vi "Configuration UI.vi"() -> ()   [LabVIEW 2012]
uses:
  cPAS.lvclass
  CRDS/Data/cCRDS Data.lvclass
  Devices/CLAP/CLAP.lvclass
  Reusable/Humidity Control/TEC/TEC Humidity Control.lvclass
  Reusable/PAS/Main/Controls/Laser Modulation.ctl
  Interface/Controls/pasLasCtl.ctl
  Interface/Controls/PAS_MFC_SP.ctl
  Interface/Controls/pasCellTEC.ctl
  Interface/Controls/pasTECen.ctl
  FPGA/Controls/FPGAConfig.ctl
panel:
  in  "ACpow":T1
  in  "pages":enum32{"general", "pas", "crds"}(tab)
  in  "pasTECEn":T2 caption="Enable TECs"
  in  "pasTcell":T3 caption="Temperature \n (degC)"
  in  "pasFlows":T4 caption="Flow Rate Setpoint (LPM)" {"Cell 5" min=0 max=5; "Cell 4" min=0 max=5; "Cell 3" min=0 max=5; "Cell 2" min=0 max=5; "Cell 1" min=0 max=5}
  in  "pasTteSP":sgl caption="TEC Temperature \nSetpoint (degC)" format="%#.2f"
  in  "pasLasCtl":T5 caption="Laser Control" {"Laser Output"."Span"."ch 5" min=0 max=20; "Laser Output"."Span"."ch 4" min=0 max=20; "Laser Output"."Span"."ch 3" min=0 max=20; "Laser Output"."Span"."ch 2" min=0 max=20; "Laser Output"."Span"."ch 1" min=0 max=20; "f0"."Cell 1" min=0 max=2000 step=1; "f0"."Cell 2" min=0 max=2000 step=1; "f0"."Cell 3" min=0 max=2000 step=1; "f0"."Cell 4" min=0 max=2000 step=1; "f0"."Cell 5" min=0 max=2000 step=1}
  # "TEC Temperature Control"
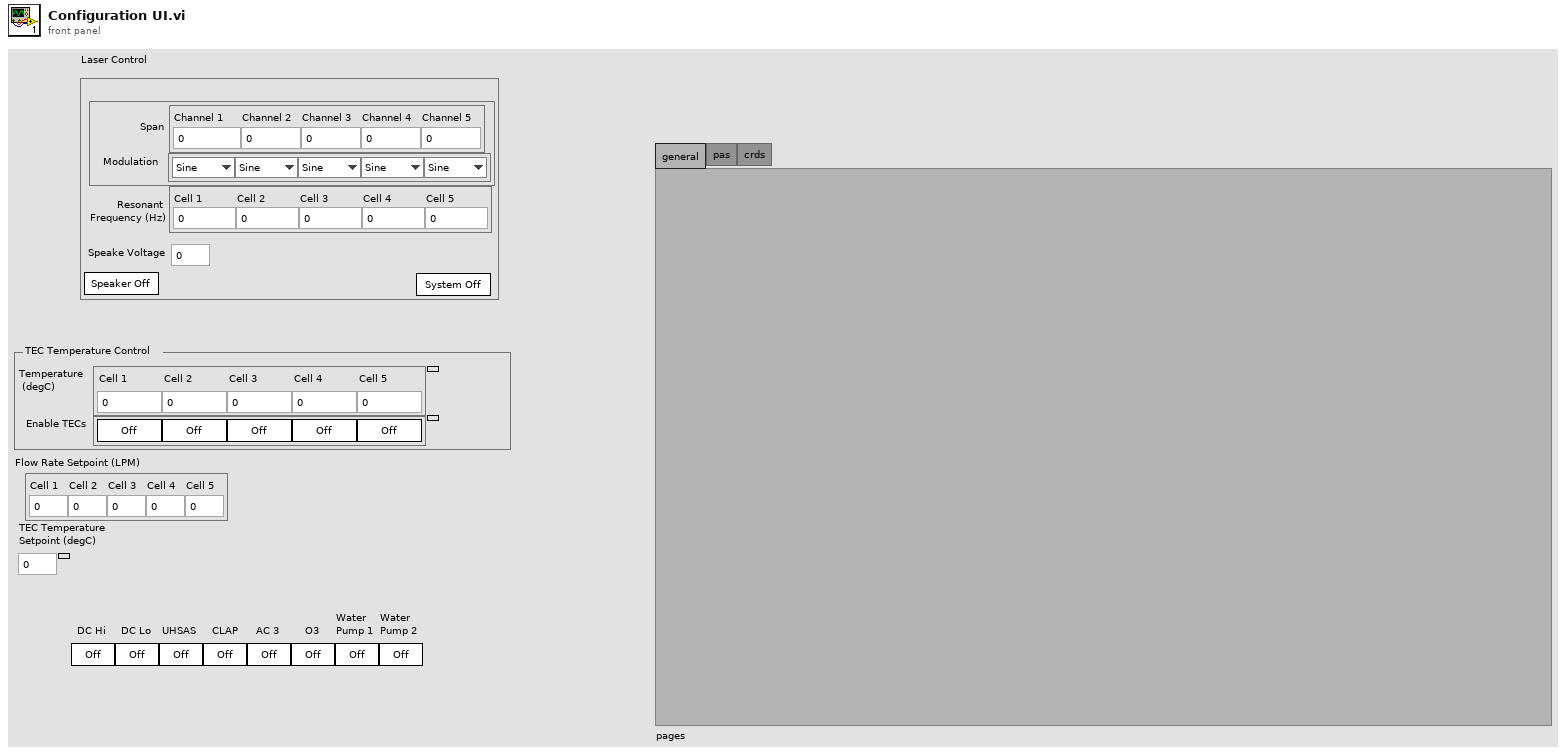
[diagram p1: front panel]
types:
  T1 = cluster{"ac1 2":bool, "ac1 3":bool, "ac1":bool, "ac2":bool, "ac3":bool, "O3":bool, "wp1":bool, "wp2":bool}
  T2 = typedef "pasTECen.ctl" = cluster{"Cell 1":bool, "Cell 2":bool, "Cell 3":bool, "Cell 4":bool, "Cell 5":bool}
  T3 = typedef "pasCellTEC.ctl" = cluster{"Cell 1":sgl, "Cell 2":sgl, "Cell 3":sgl, "Cell 4":sgl, "Cell 5":sgl}
  T4 = typedef "PAS_MFC_SP.ctl" = cluster{"Cell 1":sgl, "Cell 2":sgl, "Cell 3":sgl, "Cell 4":sgl, "Cell 5":sgl}
  T5 = typedef "pasLasCtl.ctl" = cluster{"Laser Output":T6, "f0":cluster{"Cell 1":sgl, "Cell 2":sgl, "Cell 3":sgl, "Cell 4":sgl, "Cell 5":sgl}, "drive":bool, "lasSysPow":bool, "Speake Voltage":dbl}
  T6 = typedef "FPGAConfig.ctl" = cluster{"Span":cluster{"ch 1":sgl, "ch 2":sgl, "ch 3":sgl, "ch 4":sgl, "ch 5":sgl}, "mod":cluster{"ch 1":T7, "ch 2":T7, "ch 3":T7, "ch 4":T7, "ch 5":T7}}
  T7 = typedef "Laser Modulation.ctl" = enum8{"Sine", "Square"}
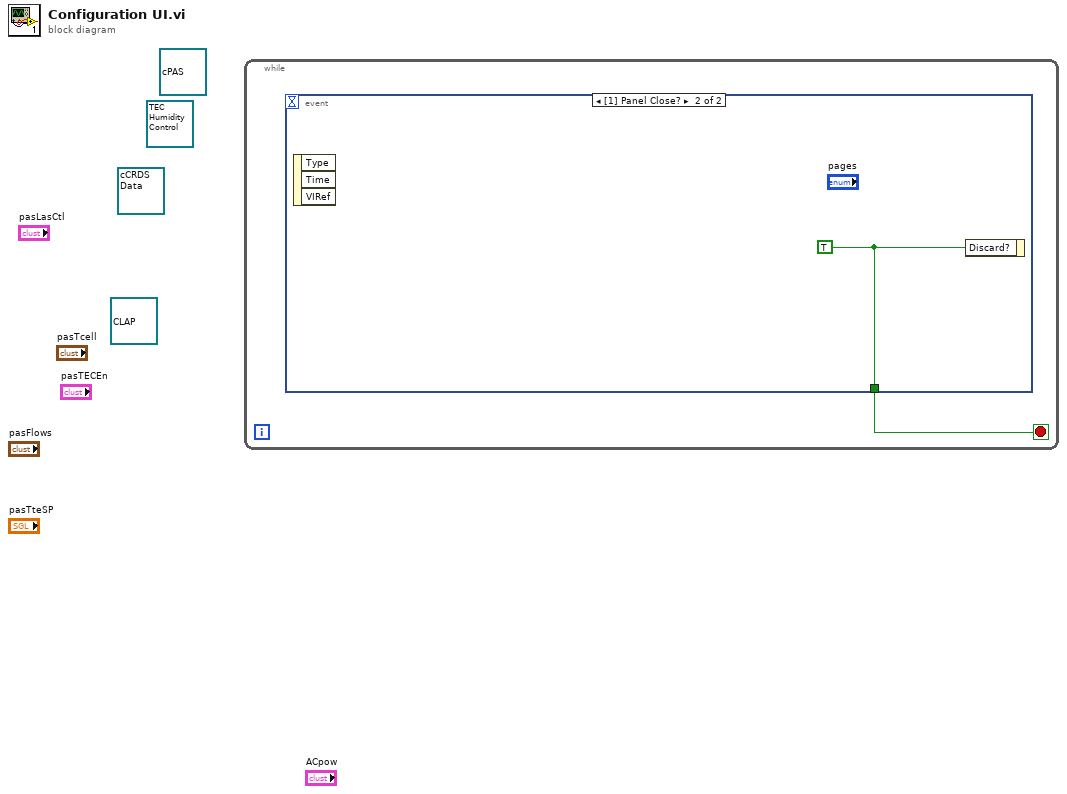
[diagram p0: block diagram]
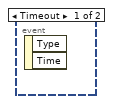
[diagram p2: hidden frame]
diagram:
  (unwired) refnum<class "TEC Humidity Control.lvclass"> refnum ("TEC Hum Ctl")
  (unwired) refnum<class "CLAP.lvclass"> refnum ("CLAP")
  (unwired) refnum<class "cCRDS Data.lvclass"> refnum ("cPAS Server Library.lvlib:cCRDS Data")
  (unwired) refnum<class "cPAS.lvclass"> refnum ("cPAS Server Library.lvlib:cPAS")
  n1 = while {
    stop <- w1 stop-if-true
    n2 = event shown="[1] Panel Close?" {
      selector: _ -> [_ _]
      dyn-events: _ -> [_ _]
      timeout: _ -> [_ _]
      tunnel: [_ w2] -> w1
      event Timeout {
        n3 = event-data() -> ()  [unwired: 1 in, 2 out]
      }
      event Panel Close? {
        w2 = TRUE ("Discard?")
        n4 = event-data() -> ()  [unwired: 1 in, 3 out]
        n5 = event-data("Discard?"=w2) -> ()  [unwired: 1 in, 1 out]
      }
    }
  }
